vi "Measure_GetData_SpectraOutput.vi"(8 "error in (no error)":errorcluster, 9 "Variant":variant, 10 "SpectraCount":i32, 11 "Avantes in":refnum<class "Avantes.lvclass">) -> (0 "error out":errorcluster, 2 "Spectra":dbl[](array[numeric]), 3 "Avantes out":refnum<class "Avantes.lvclass">, 5 "Time":dbl)   [LabVIEW 2020, in "Avantes.lvclass"]
uses:
  <instrlib>/Classes/CCD/Avantes/Avantes.lvclass
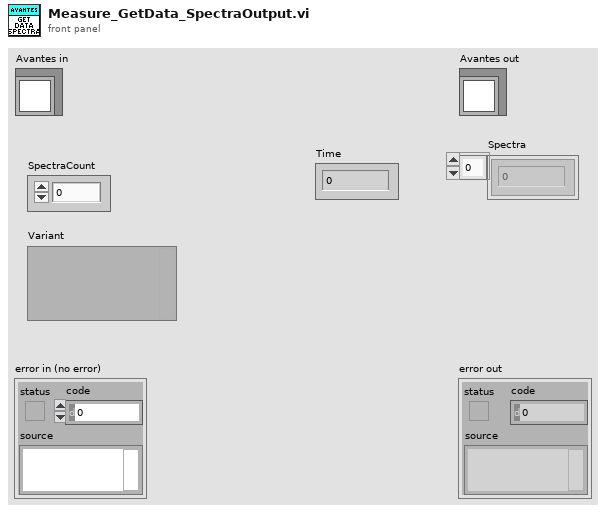
[diagram p1: front panel]
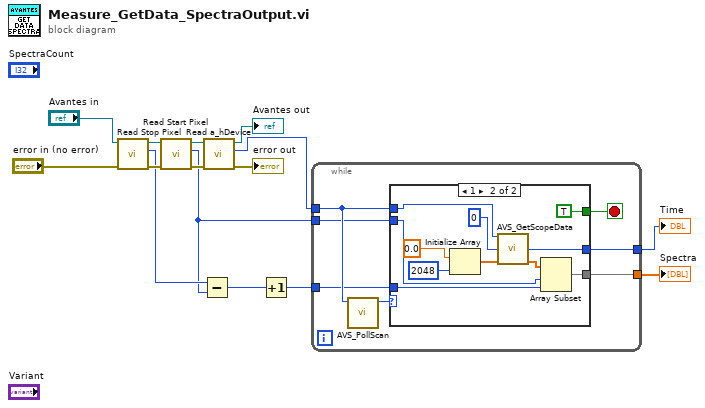
[diagram p0: block diagram]
diagram:
  n1 = call-dynamic "Read Stop Pixel.vi"("error in (no error)"="error in (no error)", "Avantes in"="Avantes in") -> ("error out"=w12:errorcluster, "Stop Pixel"=w6:u16, "Avantes out"=w11:refnum<class "Avantes.lvclass">)  [unwired: 7 in]
  n2 = call-dynamic "Read Start Pixel.vi"("error in (no error)"=w12, "Avantes in"=w11) -> ("error out"=w14:errorcluster, "Start Pixel"=w3:u16, "Avantes out"=w13:refnum<class "Avantes.lvclass">)  [unwired: 7 in]
  n3 = Subtract(x=w6, y=w3) -> (x-y=w5:u16)
  n4 = call-dynamic "Read a_hDevice.vi"("error in (no error)"=w14, "Avantes in"=w13) -> ("error out"=→"error out":errorcluster, "a_hDevice"=w15:i32, "Avantes out"=→"Avantes out":refnum<class "Avantes.lvclass">)  [unwired: 7 in]
  n5 = Increment(x=w5) -> (x+1=w4:u16)
  n6 = while {
    tunnel: w15 -> [w21]
    tunnel: [w19] -> w1
    tunnel: [w18] -> w2
    tunnel: w3 -> [w17]
    tunnel: w4 -> [w16]
    stop <- w20 stop-if-true
    n7 = call <instrlib>:"AVS_PollScan.vi"("a_hDevice"=w21) -> ("Output Value"=w22:i32)  [unwired: 8 in]
    n8 = case shown="1" w22 {
      tunnel: w21 -> [_ w30]
      tunnel: [_ TRUE] -> w20
      tunnel: [_ w28] -> w19
      tunnel: [_ w23] -> w18
      tunnel: w17 -> [_ w25]
      tunnel: w16 -> [_ w24]
      frame 0, Default {
      }
      frame 1 {
        n9 = Initialize Array(0.0 ("element"), 2048 ("dimension size")) -> (w32:dbl[])
        n10 = call <instrlib>:"AVS_GetScopeData.vi"("a_hDevice"=w30, "a_pTimeLabel"=u32 0, "a_pSpectrum"=w32) -> ("a_pTimeLabel"=w28:u32, "a_pSpectrum"=w26:dbl[])  [unwired: 10 in, 1 out]
        n11 = Array Subset(array=w26, index=w25, length=w24) -> (w23:dbl[])
      }
    }
  }
  "Spectra" <- w2
  "Time" <- w1
